vi "uDAQbinaryParser.vi"(7 "FS Range":sgl, 9 "DataLength":i32=128, 10 "DataStart":i32=3, 11 "ByteArray":u8[](array[numeric])=array[5000 elements]) -> (3 "Data":dbl[](array[numeric]))   [LabVIEW 2017]
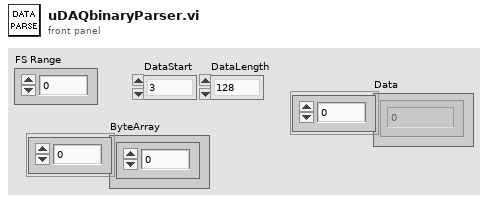
[diagram p1: front panel]
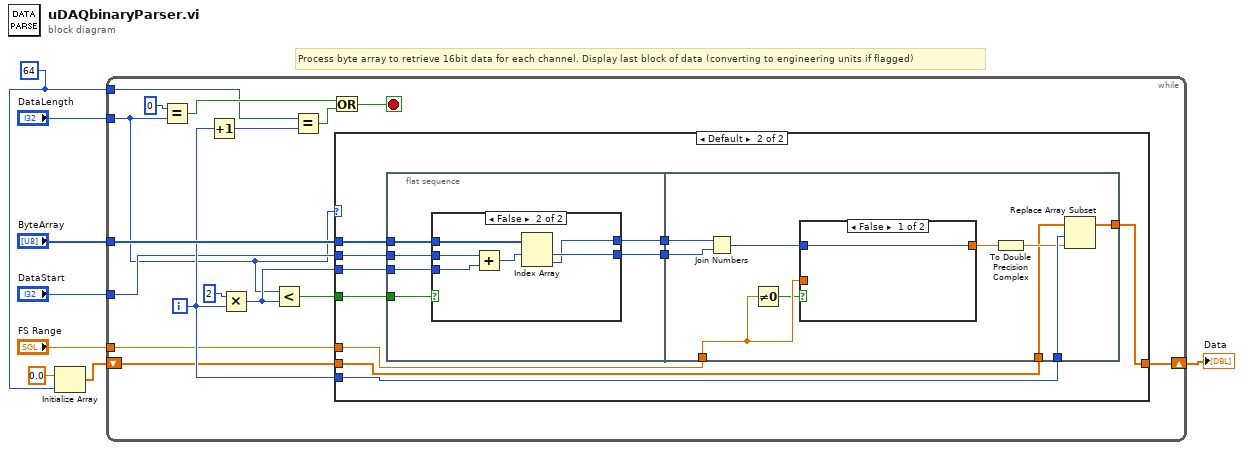
[diagram p0: block diagram]
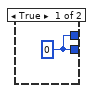
[diagram p3: hidden frame]
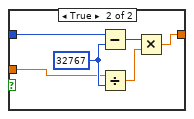
[diagram p4: hidden frame]
diagram:
  w3 = 64 ("x")
  # "Process byte array to retrieve 16bit data for each channel. Display last block of data (converting to engineering units if flagged)"
  n1 = Initialize Array(0.0 ("element"), w3) -> (w1:dbl[])
  n2 = while {
    tunnel: "ByteArray" -> [w23]
    tunnel: "DataStart" -> [w14]
    tunnel: "DataLength" -> [w13]
    tunnel: "FS Range" -> [w12]
    shift-right: [w11] -> w4
    shift-left: w1 -> [w10]
    tunnel: w3 -> [w9]
    i -> [w17]
    stop <- w20 stop-if-true
    n3 = Equal?(x=u8 0, y=w13) -> (x = y?=w21:bool)
    n4 = Increment(x=w17) -> (x+1=w16:i32)
    n5 = Multiply(x=u8 2, y=w17) -> (x*y=w22:i32)
    n6 = Less?(x=w13, y=w22) -> (x < y?=w18:bool)
    n7 = Equal?(x=w9, y=w16) -> (x = y?=w15:bool)
    n8 = Or(x=w21, y=w15) -> (x .or. y?=w20:bool)
    n9 = case shown="Default" w13 {
      tunnel: w23 -> [_ w35]
      tunnel: w22 -> [_ w34]
      tunnel: w17 -> [_ w32]
      tunnel: w18 -> [_ w33]
      tunnel: w14 -> [_ w31]
      tunnel: w12 -> [_ w28]
      tunnel: [w25 w27] -> w11
      tunnel: w10 -> [w25 w26]
      frame 0 {
      }
      frame Default {
        n10 = flat-sequence {
          tunnel: w35 -> [w41]
          tunnel: w34 -> [w40]
          tunnel: w33 -> [w39]
          tunnel: w31 -> [w38]
          tunnel: [w37] -> w30
          tunnel: [w36] -> w29
          tunnel: w32 -> [w54]
          tunnel: w30 -> [w56]
          tunnel: w29 -> [w55]
          tunnel: w28 -> [w50]
          tunnel: [w52] -> w27
          tunnel: w26 -> [w51]
          frame #0 {
            n11 = case shown="False" w39 {
              tunnel: w41 -> [_ w46]
              tunnel: w40 -> [_ w48]
              tunnel: w38 -> [_ w47]
              tunnel: [w42 w44] -> w37
              tunnel: [w42 w43] -> w36
              frame True {
                w42 = u8 0
              }
              frame False {
                n12 = Add(x=w47, y=w48) -> (x+y=w45:i32)
                n13 = Index Array(array=w46, index #1=w45) -> (element #1=w44:u8, element #2=w43:u8)  [unwired: 1 in]
              }
            }
          }
          frame #1 {
            n14 = Join Numbers(hi=w55, lo=w56) -> ((hi.lo)=w58:u16)
            n15 = Not Equal To 0?(x=w50) -> (x != 0?=w49:bool)
            n16 = case shown="False" w49 {
              tunnel: w58 -> [w59 w65]
              tunnel: [w59 w61] -> w57
              tunnel: w50 -> [_ w60]
              frame False {
              }
              frame True {
                w64 = 32767
                n17 = Subtract(x=w65, y=w64) -> (x-y=w63:i32)
                n18 = Divide(x=w60, y=w64) -> (x/y=w62:sgl)
                n19 = Multiply(x=w63, y=w62) -> (x*y=w61:sgl)
              }
            }
            n20 = To Double Precision Complex(1:w57) -> (0:w53:cdb)
            n21 = Replace Array Subset(array=w51, new element=w53, index=w54) -> (w52:dbl[])
          }
        }
      }
    }
  }
  "Data" <- w4
